vi "Update Nested Message.vi"(8 "error in (no error)":errorcluster, 10 "Message":string, 11 "Root in":refnum<class "Root.lvclass">) -> (0 "error out":errorcluster, 3 "Root out":refnum<class "Root.lvclass">)   [LabVIEW 2025, in "Root.lvlib" / "Root.lvclass"]
uses:
  Root.lvclass
  Root.lvclass/Root.ctl
  Nested/Nested Messages/Update Message from Root Msg/Update Message from Root Msg.lvclass/Update Message from Root Msg.ctl
  <vilib>/ActorFramework/Message Enqueuer/Message Enqueuer.lvclass/Message Enqueuer.ctl
  <vilib>/ActorFramework/Message Enqueuer/Enqueue.vi
  Nested/Nested Messages/Update Message from Root Msg/Update Message from Root Msg.lvclass
  C:/Program Files/National Instruments/LabVIEW 2025/vi.lib/ActorFramework/Message/Message.lvclass
  <vilib>/ActorFramework/Message Priority Queue/Priority Enqueue.vi
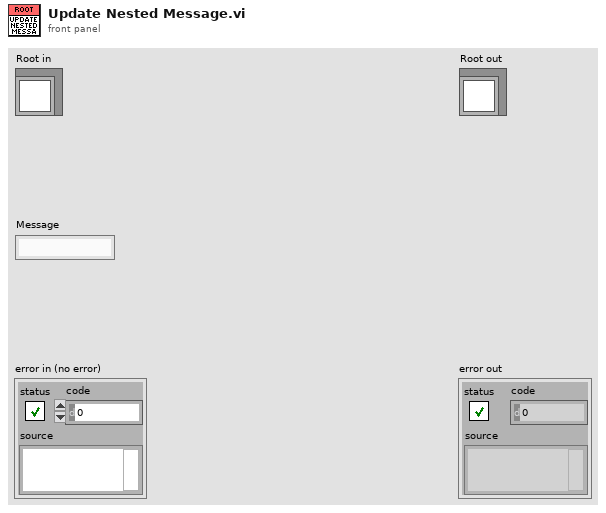
[diagram p1: front panel]
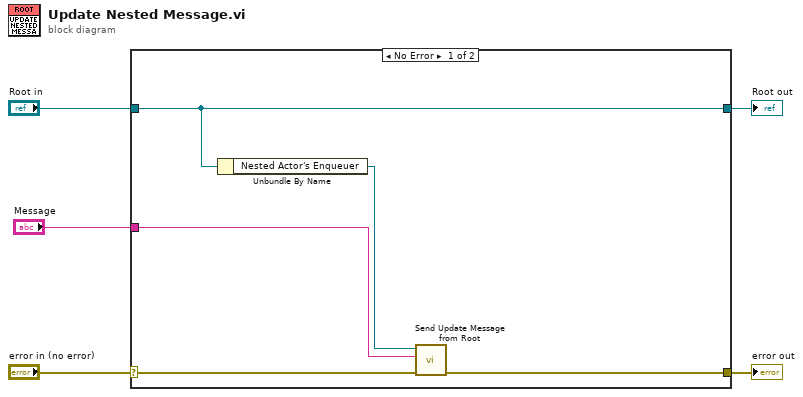
[diagram p0: block diagram]
diagram:
  n1 = case shown="No Error" "error in (no error)" {
    selector: "error in (no error)" -> [w8 w12]
    tunnel: [w9 w12] -> w4
    tunnel: [w10 w11] -> w2
    tunnel: "Root in" -> [w10 w11]
    tunnel: "Message" -> [w6 _]
    frame No Error {
      n2 = Unbundle By Name(w10) -> ("Nested Actor's Enqueuer"=w7:refnum<class "Message Enqueuer.lvclass">)
      n3 = call "Send Update Message from Root.vi"("error in (no error)"=w8, "Message"=w6, "Message Enqueuer"=w7) -> ("error out"=w9:errorcluster)  [unwired: 7 in, 1 out]
    }
    frame Error {
    }
  }
  "error out" <- w4
  "Root out" <- w2
